vi "Add Server Certificate Paths.vi"(10 "Server Connection Configuration In":T1) -> (2 "Server Connection Configuration Out":T1)   [LabVIEW 2013, in "OPC UA Client Tests.lvlib"]
doc: "Add Certificate paths to Server configuration"
uses:
  OPC UA Client Tests.lvlib
  Server Connection Configuration.ctl
  <vilib>/OPCUA/server/subVI/supported security policies.ctl
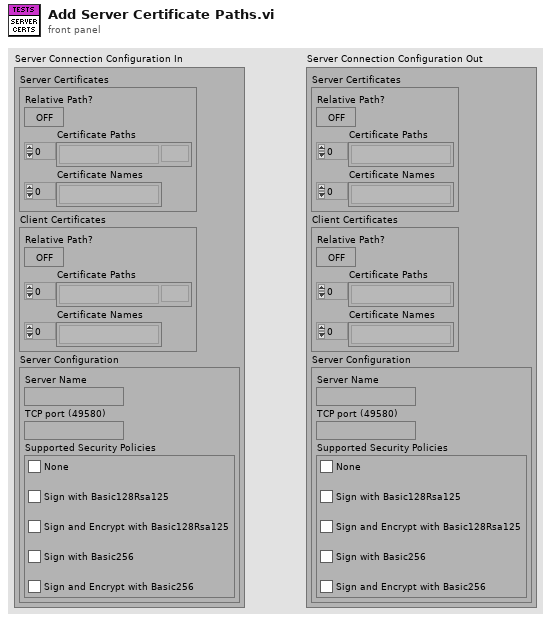
[diagram p1: front panel]
types:
  T1 = typedef "OPC UA Client Tests.lvlib/Server Connection Configuration.ctl" = cluster{"Server Certificates":cluster{"Relative Path?":bool, "Certificate Paths":path[], "Certificate Names":string[]}, "Client Certificates":cluster{"Relative Path?":bool, "Certificate Paths":path[], "Certificate Names":string[]}, "Server Configuration":cluster{"Server Name":string, "TCP port (49580)":string, "Supported Security Policies":T2}}
  T2 = typedef "supported security policies.ctl" = cluster{"None":bool, "Sign with Basic128Rsa125":bool, "Sign and Encrypt with Basic128Rsa125":bool, "Sign with Basic256":bool, "Sign and Encrypt with Basic256":bool}
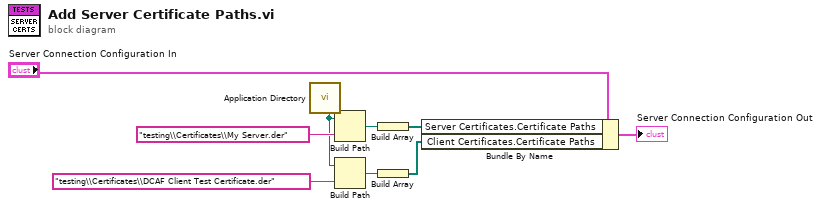
[diagram p0: block diagram]
diagram:
  n1 = call <vilib>:"Application Directory.vi"() -> ("Application Directory"=w3:path)
  n2 = Build Path(base path=w3, name or relative path="testing\\Certificates\\My Server.der") -> (appended path=w6:path)
  n3 = Build Path(base path=w3, name or relative path="testing\\Certificates\\DCAF Client Test Certificate.der") -> (appended path=w8:path)
  n4 = Build Array(w6) -> (w7:path[])
  n5 = Build Array(w8) -> (w9:path[])
  n6 = Bundle By Name(cluster="Server Connection Configuration In", "Server Certificates.Certificate Paths"=w7, "Client Certificates.Certificate Paths"=w9) -> (→"Server Connection Configuration Out":T1)
